vi "Plot Default Sine Cos Graph with Write Delimited Spreadsheet with delimiter csv.vi"() -> ()   [LabVIEW 2020]
uses:
  <vilib>/Utility/file.llb/Write Delimited Spreadsheet (DBL).vi
panel:
  out "Data":dbl[](array[numeric])
  out "Waveform Graph":dbl[][](graph)
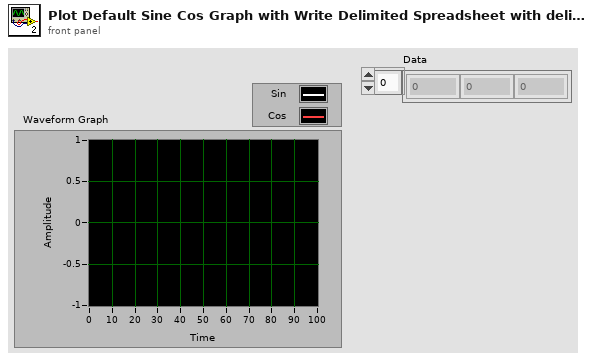
[diagram p1: front panel]
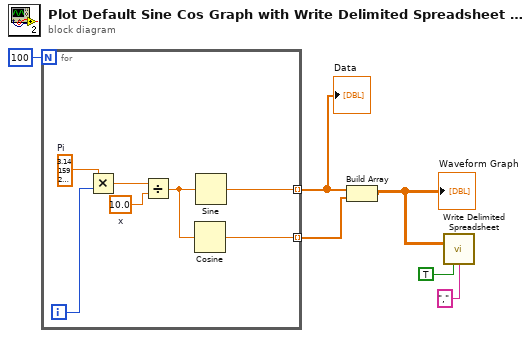
[diagram p0: block diagram]
diagram:
  n1 = for {
    N: 100 -> [_]
    tunnel: [w9] -> w5 mode=indexing
    tunnel: [w7] -> w4 mode=indexing
    i -> [w13]
    w10 = 10.0  # x
    w12 = 3.141592653589793  # Pi
    n2 = Multiply(x=w12, y=w13) -> (x*y=w11:dbl)
    n3 = Divide(x=w11, y=w10) -> (x/y=w8:dbl)
    n4 = Cosine(x=w8) -> (cos(x)=w7:dbl)
    n5 = Sine(x=w8) -> (sin(x)=w9:dbl)
  }
  "Data" <- w5
  n6 = Build Array(w5, w4) -> (w3:dbl[][])
  "Waveform Graph" <- w3
  n7 = call-poly <vilib>:"Write Delimited Spreadsheet.vi"("2D data"=w3, "transpose? (no:F)"=TRUE, "delimiter (\\t)"="," ("delimiter (\\t)")) -> ()  [unwired: 11 in, 2 out]
